vi "Uninit.vi"(11 "Supervisor in":refnum<class "Supervisor.lvclass">) -> (3 "Supervisor out":refnum<class "Supervisor.lvclass">)   [LabVIEW 2020, in "Supervisor.lvlib" / "Supervisor.lvclass"]
doc: "This method is the inverse of the Pre Launch Init.vi. This method is called unconditionally at the end of an actor's lifetime, even if there was an error in Pre Launch Init.vi. Note that the self Enqueuer for the actor is already invalid by the time this VI executes: within this method, the actor may send messages to its caller but not to itself. This method executes before Last Ack is sent.\n\nThis method neither receives nor produces an error cluster. It is designed to provide an unconditional release of acquired resources. Any error raised during release is considered to be irrelevant to the actor's lifetime. If the actor truly needs to report some error status, it may send a message to caller or include information within itself that callers can examine when handling Last Ack."
uses:
  Supervisor.lvclass
  Supervisor.lvclass/Supervisor.ctl
  <vilib>/ActorFramework/Actor/Actor.lvclass
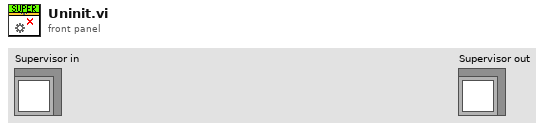
[diagram p1: front panel]
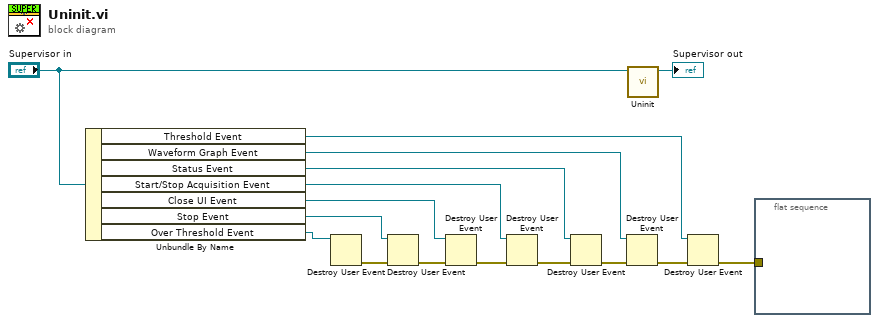
[diagram p0: block diagram]
diagram:
  n1 = Unbundle By Name("Supervisor in") -> ("Threshold Event"=w8:refnum<user-event>, "Waveform Graph Event"=w7:refnum<user-event>, "Status Event"=w6:refnum<user-event>, "Start/Stop Acquisition Event"=w5:refnum<user-event>, "Close UI Event"=w4:refnum<user-event>, "Stop Event"=w3:refnum<user-event>, "Over Threshold Event"=w2:refnum<user-event>)
  n2 = Destroy User Event(user event=w2) -> (error out=w1:errorcluster)  [unwired: 1 in]
  n3 = Destroy User Event(user event=w3, error in=w1) -> (error out=w11:errorcluster)
  n4 = Destroy User Event(user event=w4, error in=w11) -> (error out=w15:errorcluster)
  n5 = Destroy User Event(user event=w5, error in=w15) -> (error out=w14:errorcluster)
  n6 = Destroy User Event(user event=w6, error in=w14) -> (error out=w13:errorcluster)
  n7 = Destroy User Event(user event=w7, error in=w13) -> (error out=w12:errorcluster)
  n8 = call-parent "Uninit.vi"("Actor in"="Supervisor in") -> ("Actor out"=→"Supervisor out":refnum<class "Supervisor.lvclass">)  [unwired: 10 in]
  n9 = Destroy User Event(user event=w8, error in=w12) -> (error out=w10:errorcluster)
  n10 = flat-sequence {
    tunnel: w10 -> [_]
    frame #0 {
    }
  }
